vi "heron.vi"(8 "error in":errorcluster, 9 "c":dbl=5.0, 10 "b":dbl=4.0, 11 "a":dbl=3.0) -> (0 "error out":errorcluster, 3 "area":dbl)   [LabVIEW 2024]
doc: "Calculatess the area of triangle"
uses:
  <vilib>/Utility/error.llb/Error Cluster From Error Code.vi
  <vilib>/ErrorRing/Error Ring.xnode
panel:
  out "areaSquared":dbl
  out "p":dbl
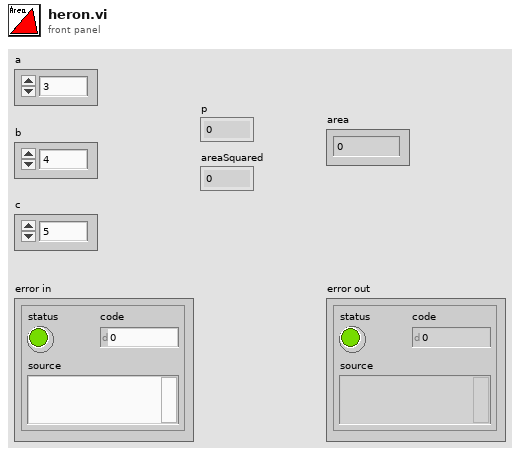
[diagram p1: front panel]
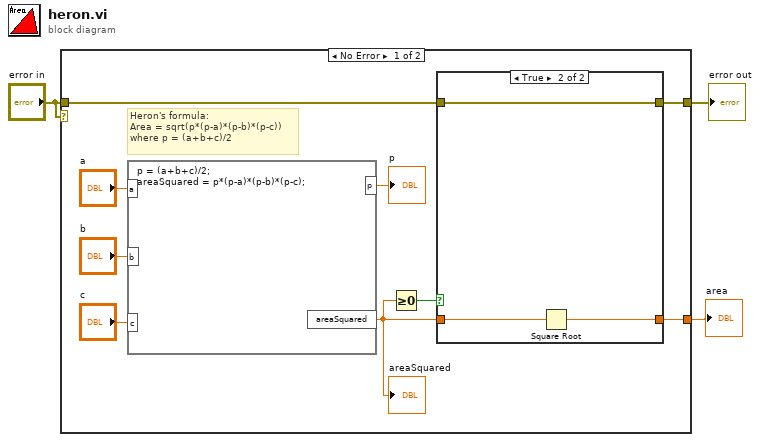
[diagram p0: block diagram]
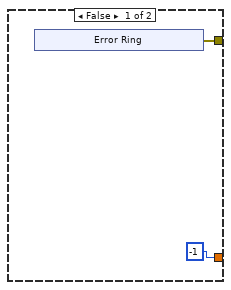
[diagram p2: hidden frame]
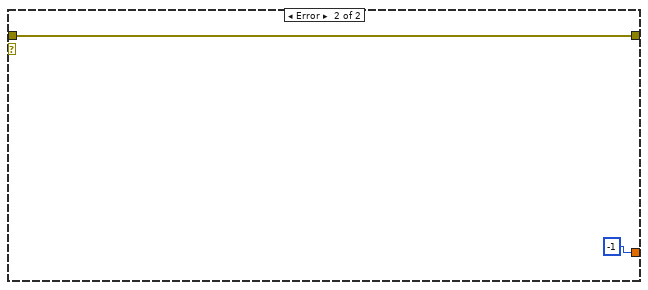
[diagram p3: hidden frame]
diagram:
  n1 = case shown="No Error" "error in" {
    tunnel: "error in" -> [w4 w23]
    tunnel: [w6 -1] -> w3
    tunnel: [w5 w23] -> w1
    frame No Error {
      # "Heron's formula:\nArea = sqrt(p*(p-a)*(p-b)*(p-c))\nwhere p = (a+b+c)/2"
      n2 = formula code="p = (a+b+c)/2;\nareaSquared = p*(p-a)*(p-b)*(p-c);"("a"="a", "b"="b", "c"="c") -> ("p"=→"p":dbl, "areaSquared"=w12:dbl)
      "areaSquared" <- w12
      n3 = Greater Or Equal To 0?(x=w12) -> (x >= 0?=w11:bool)
      n4 = case shown="True" w11 {
        tunnel: [w13 w20] -> w5
        tunnel: w12 -> [_ w22]
        tunnel: [-1 w21] -> w6
        tunnel: w4 -> [_ w20]
        frame False {
          n5 = xnode "Error Ring"() -> ("error out"=w13:errorcluster)
        }
        frame True {
          n6 = Square Root(x=w22) -> (sqrt(x)=w21:dbl)
        }
      }
    }
    frame Error {
    }
  }
  "error out" <- w1
  "area" <- w3
